vi "SetGainSpeed.vi"(1 "Gain":i32=1 min=1 max=10) -> (0 "Error":bool)   [LabVIEW 2014]
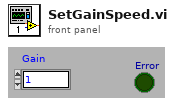
[diagram p1: front panel]
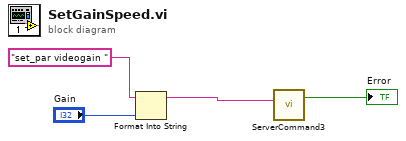
[diagram p0: block diagram]
diagram:
  n1 = Format Into String(initial string="set_par videogain " ("Command"), "Gain") -> (resulting string=w1:string)  [unwired: 2 in, 1 out]
  n2 = call "ServerCommand3.vi"("Command"=w1) -> ("Error"=→"Error":bool)  [unwired: 1 out]
